vi "trigger-test4.vi"() -> ()   [LabVIEW 2020]
uses:
  Realization/PI650 VoltageAmp/TypeDefs/Channel gain.ctl
  Realization/PIPX40 Matrix/PIPX40 Matrix.lvclass
  Realization/PI650 VoltageAmp/PI650 VoltageAmp.lvclass
  Realization/PI650 VoltageAmp/TypeDefs/Channel DC offset.ctl
  Realization/NI PXI Trigger/NI PXI Trigger.lvclass
  Realization/NI PXI Trigger/PXI Trigger config.ctl
  Realization/NI DMM/NI DMM.lvclass
  Realization/NI DMM/TypeDefs/DMM waveform settings.ctl
  <instrlib>/niDMM/nidmm.llb/niDMM Waveform Function.ctl
  Realization/NI DMM/TypeDefs/Trigger settings.ctl
  <instrlib>/niDMM/nidmm.llb/niDMM Trigger.ctl
  <instrlib>/niDMM/nidmm.llb/niDMM Slope.ctl
  Realization/NI Analog Input/NI Analog Input.lvclass
  Realization/NI DAQmx Base/TypeDefs/Channel Config.ctl
  Realization/NI Analog Output/TypeDefs/Timing Config.ctl
  Realization/NI Analog Output/TypeDefs/Trigger Config.ctl
  Realization/NI Analog Output/NI Analog Output.lvclass
  <instrlib>/niDCPower/nidcpower.llb/niDCPower Output Function.ctl
  Realization/PIPX40 Relay/PIPX40 Relay.lvclass
  <vilib>/measure/NI_MABase.lvlib
panel:
  out "relay info":variant
  out "current measurements":dbl[](array[numeric])
  out "voltage measurements":dbl[](array[numeric])
  in  "instrument handle":refnum<k15>="NI_SMU1"
  in  "noise level":dbl=0.05 format="%#_3f"
  in  "signal type":T1(ring)
  in  "Channel gain":T2={"Channel (CH1)"=3, "Gain (x1)"=2} {"Channel (CH1)" items=["CH1"=1, "CH2"=2, "CH3"=3, "CH4"=4, "CH5"=5]; "Gain (x1)" items=["x1"=1, "x2"=2, "x5"=3, "x7"=4, "x10"=5, "x14"=6, "x20"=7]}
  out "Amp Info":variant
  out "Mx infos":variant[](array[variant])
  out "Waveform Graph":dynamicdata(graph)
  out "error out":errorcluster
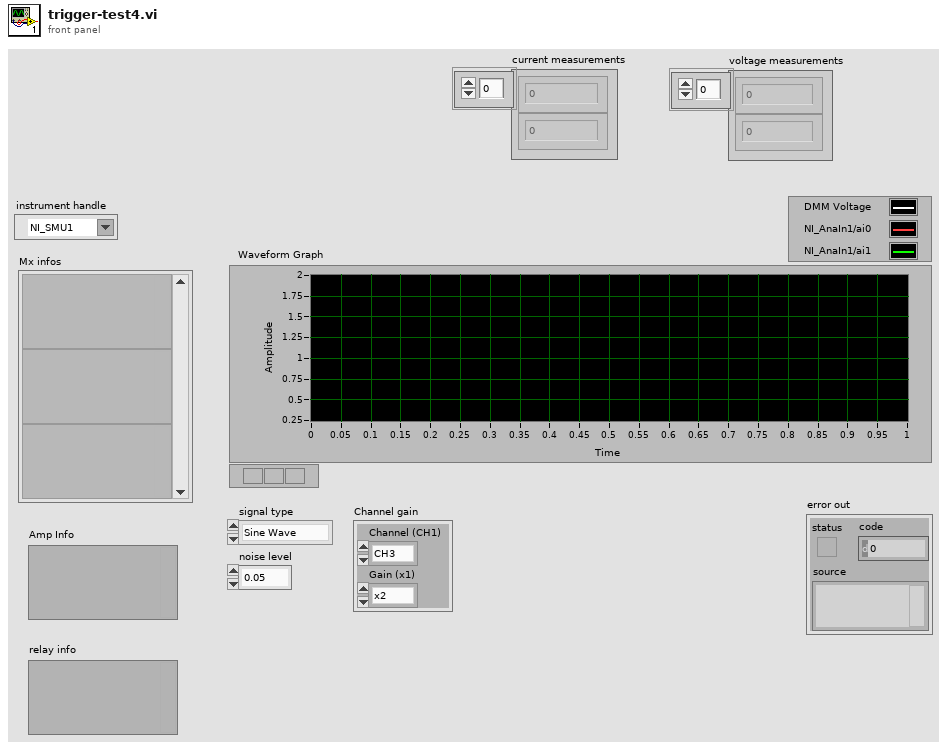
[diagram p1: front panel]
types:
  T1 = enum16{"Sine Wave", "Triangle Wave", "Square Wave", "Sawtooth Wave"}
  T2 = typedef "Channel gain.ctl" = cluster{"Channel (CH1)":u32, "Gain (x1)":u32}
  T3 = typedef "niDCPower Output Function.ctl" = i32
  T4 = typedef "Trigger Config.ctl" = cluster{"trigger type":string, "source":string, "slope":i32, "analog level":dbl, "analog hysteresis":dbl}
  T5 = typedef "Timing Config.ctl" = cluster{"sample mode":i32, "samples per channel":i32, "rate":dbl, "source":string, "active edge":i32}
  T6 = typedef "Channel Config.ctl" = cluster{"channels":string, "maximum value":dbl, "minimum value":dbl, "output terminal configuration":i32, "units":i32}
  T7 = typedef "Trigger settings.ctl" = cluster{"Trigger Source":T8, "Trigger Delay (sec)":dbl, "Slope":T9}
  T8 = typedef "niDMM Trigger.ctl" = enum16{"Immediate", "External", "TTL 0", "TTL 1", "TTL 2", "TTL 3", "TTL 4", "TTL 5", "TTL 6", "Software", "TTL 7", "PXI Star", "LBR Trig 1", "Aux Trig 1"}
  T9 = typedef "niDMM Slope.ctl" = enum16{"Rising Edge", "Falling Edge"}
  T10 = typedef "DMM waveform settings.ctl" = cluster{"Waveform Points":i32, "Function":T11, "Rate":dbl, "Range":dbl, "Settle Time":dbl}
  T11 = typedef "niDMM Waveform Function.ctl" = i32
  T12 = typedef "PXI Trigger config.ctl" = cluster{"counter output":string, "source terminal":string, "destination terminal":string}
  T13 = typedef "Channel DC offset.ctl" = cluster{"Channel (CH1)":u32, "Offset (128)":u32}
  T14 = map{string, refnum<class "PIPX40 Matrix.lvclass">}
  T15 = cluster{"samples per channel":dbl, "samples per channel":dbl}
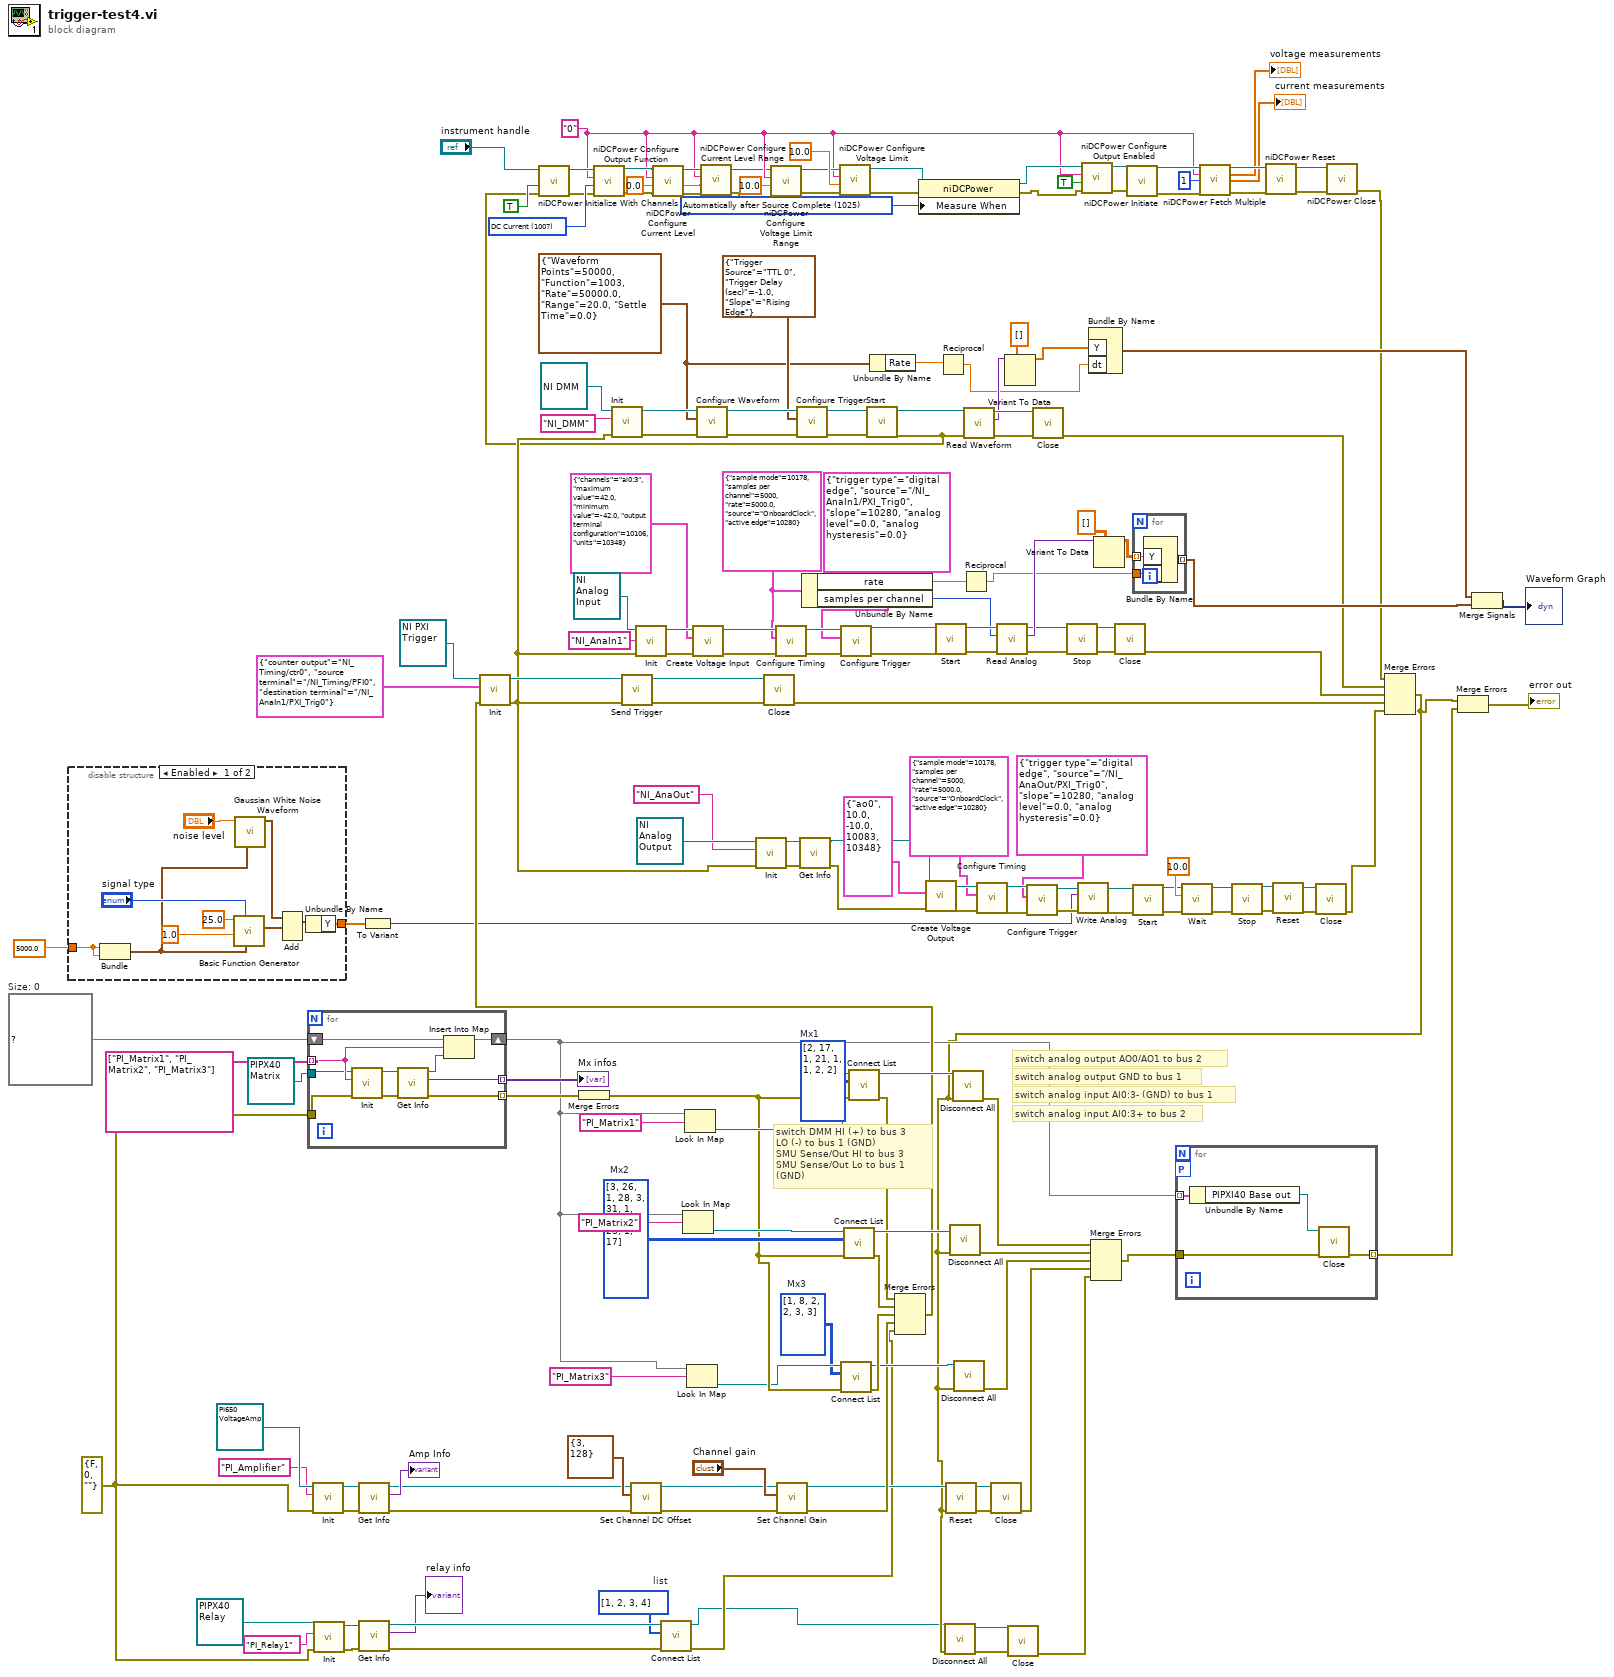
[diagram p0: block diagram]
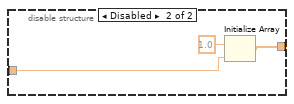
[diagram p2: hidden frame]
diagram:
  w6 = i32[] [1, 2, 3, 4]  # list
  w26 = 1025 items=["Automatically after Source Complete"=1025, "On Demand"=1026, "On Measure Trigger"=1027] ("Measurement:Advanced:Measure When")
  w18 = 0.0 ("current level")
  w19 = "0" ("channel name")
  w50 = T3 1007 items=["DC Voltage"=1006, "DC Current"=1007, "Pulse Voltage"=1049, "Pulse Current"=1050] ("output function")
  w83 = T5 {"sample mode"=10178, "samples per channel"=5000, "rate"=5000.0, "source"="OnboardClock", "active edge"=10280}
  w111 = T10 {"Waveform Points"=50000, "Function"=1003, "Rate"=50000.0, "Range"=20.0, "Settle Time"=0.0}
  w5 = errorcluster {"status"=FALSE, "code"=0, "source"=""} ("error in (no error)")
  w153 = i32[][] [[1, 8], [2, 2], [3, 3]]  # Mx3
  w164 = T14 {}  # Size: 0
  w173 = i32[][] [[3, 26], [1, 28], [3, 31], [1, 19], [3, 23], [1, 17]]  # Mx2
  w175 = i32[][] [[2, 17], [1, 21], [1, 1], [2, 2]]  # Mx1
  # "switch analog input AI0:3+ to bus 2"
  # "switch analog input AI0:3- (GND) to bus 1"
  # "switch analog output GND to bus 1"
  # "switch analog output AO0/AO1 to bus 2"
  # "switch DMM HI (+) to bus 3 \nLO (-) to bus 1 (GND)\nSMU Sense/Out HI to bus 3\nSMU Sense/Out Lo to bus 1 (GND)"
  n1 = disable-structure shown="Enabled" {
    disable-tunnel: 5000.0 ("samples per channel") -> [w189 w192]
    disable-tunnel: [w188 w194] -> w133
    frame Enabled {
      n2 = Bundle("samples per channel"=w189, "samples per channel"=w189) -> (w186:T15)  [unwired: 1 in]
      n3 = call <vilib>:"Basic Function Generator.vi"("sampling info"=w186, "signal type"="signal type", "amplitude"=1.0, "frequency"=25.0) -> ("signal out"=w185:waveform(dbl))  [unwired: 5 in, 2 out]
      n4 = call <vilib>:"Gaussian White Noise Waveform.vi"("sampling info"=w186, "standard deviation"="noise level") -> ("signal out"=w184:waveform(dbl))  [unwired: 8 in, 1 out]
      n5 = Add(1:w185, 2:w184) -> (0:w183:waveform(dbl))  [unwired: 1 in, 1 out]
      n6 = Unbundle By Name(w183) -> ("Y"=w188:dbl[])
    }
    frame Disabled {
      n7 = Initialize Array(1.0 ("element"), w192) -> (w194:dbl[])
    }
  }
  n8 = for {
    tunnel: string[] ["PI_Matrix1", "PI_Matrix2", "PI_Matrix3"] -> [w200] mode=indexing
    tunnel: [w203] -> w178 mode=indexing
    tunnel: [w202] -> w177 mode=indexing
    shift-right: [w201] -> w156
    shift-left: w164 -> [w198]
    tunnel: refnum<class "PIPX40 Matrix.lvclass"> refnum ("PIPXI40 Matrix in") -> [w196]
    tunnel: w5 -> [w195]
    n9 = call-dynamic "Init.vi"("error in (no error)"=w195, "Params"=w200, "PIPXI40 Base in"=w196) -> ("error out"=w204:errorcluster, "PIPXI40 Base out"=w199:refnum<class "PIPX40 Matrix.lvclass">)  [unwired: 7 in]
    n10 = call-dynamic "Get Info.vi"("error in (no error)"=w204, "PIPXI40 Base in"=w199) -> ("error out"=w203:errorcluster, "Info"=w202:variant, "PIPXI40 Base out"=w197:refnum<class "PIPX40 Matrix.lvclass">)  [unwired: 7 in]
    n11 = Insert Into Map(map in=w198, key=w200, value=w197) -> (map out=w201:T14)  [unwired: 2 out]
  }
  "Mx infos" <- w177
  n12 = call-dynamic "Init.vi"("error in (no error)"=w5, "Params"="PI_Amplifier" ("String"), "PI650 VoltageAmp in"=refnum<class "PI650 VoltageAmp.lvclass"> refnum) -> ("error out"=w147:errorcluster, "PI650 VoltageAmp out"=w148:refnum<class "PI650 VoltageAmp.lvclass">)  [unwired: 7 in]
  n13 = call-dynamic "Init.vi"("error in (no error)"=w5, "Params"="PI_Relay1" ("String"), "PIPXI40 Base in"=refnum<class "PIPX40 Relay.lvclass"> refnum ("Pickering.lvlib:PIPX40 Relay.lvclass")) -> ("error out"=w15:errorcluster, "PIPXI40 Base out"=w12:refnum<class "PIPX40 Relay.lvclass">)  [unwired: 7 in]
  n14 = call-dynamic "Get Info.vi"("error in (no error)"=w147, "PI650 VoltageAmp in"=w148) -> ("error out"=w142:errorcluster, "Info"=→"Amp Info":variant, "PI650 VoltageAmp out"=w141:refnum<class "PI650 VoltageAmp.lvclass">)  [unwired: 7 in]
  n15 = call-dynamic "Get Info.vi"("error in (no error)"=w15, "PIPXI40 Base in"=w12) -> ("error out"=w9:errorcluster, "Info"=→"relay info":variant, "PIPXI40 Base out"=w11:refnum<class "PIPX40 Relay.lvclass">)  [unwired: 7 in]
  n16 = To Variant(anything=w133) -> (Variant=w53:variant)
  n17 = Merge Errors(w178) -> (w155:errorcluster)
  n18 = call-dynamic "Set Channel DC Offset.vi"("error in (no error)"=w142, "Params"=T13 {"Channel (CH1)"=3, "Offset (128)"=128}, "PI650 VoltageAmp in"=w141) -> ("error out"=w139:errorcluster, "PI650 VoltageAmp out"=w140:refnum<class "PI650 VoltageAmp.lvclass">)  [unwired: 7 in]
  n19 = call-dynamic "Connect List.vi"("error in (no error)"=w9, "Params"=w6, "PIPXI40 Switching in"=w11) -> ("error out"=w2:errorcluster, "PIPXI40 Switching out"=w1:refnum<class "PIPX40 Relay.lvclass">)  [unwired: 7 in]
  n20 = Look In Map(map=w156, key="PI_Matrix2" ("String")) -> (value=w166:refnum<class "PIPX40 Matrix.lvclass">)  [unwired: 1 in, 1 out]
  n21 = Look In Map(map=w156, key="PI_Matrix1" ("String")) -> (value=w167:refnum<class "PIPX40 Matrix.lvclass">)  [unwired: 1 in, 1 out]
  n22 = Look In Map(map=w156, key="PI_Matrix3" ("String")) -> (value=w154:refnum<class "PIPX40 Matrix.lvclass">)  [unwired: 1 in, 1 out]
  n23 = call-dynamic "Set Channel Gain.vi"("error in (no error)"=w139, "Params"="Channel gain", "PI650 VoltageAmp in"=w140) -> ("error out"=w138:errorcluster, "PI650 VoltageAmp out"=w135:refnum<class "PI650 VoltageAmp.lvclass">)  [unwired: 7 in]
  n24 = Unbundle By Name(w83) -> ("rate"=w81:dbl, "samples per channel"=w82:i32)
  n25 = call-dynamic "Connect List.vi"("error in (no error)"=w155, "Params"=w153, "PIPXI40 Matrix in"=w154) -> ("error out"=w152:errorcluster, "PIPXI40 Matrix out"=w151:refnum<class "PIPX40 Matrix.lvclass">)  [unwired: 7 in]
  n26 = call-dynamic "Connect List.vi"("error in (no error)"=w155, "Params"=w173, "PIPXI40 Matrix in"=w166) -> ("error out"=w162:errorcluster, "PIPXI40 Matrix out"=w171:refnum<class "PIPX40 Matrix.lvclass">)  [unwired: 7 in]
  n27 = call-dynamic "Connect List.vi"("error in (no error)"=w155, "Params"=w175, "PIPXI40 Matrix in"=w167) -> ("error out"=w163:errorcluster, "PIPXI40 Matrix out"=w172:refnum<class "PIPX40 Matrix.lvclass">)  [unwired: 7 in]
  n28 = Unbundle By Name(w111) -> ("Rate"=w110:dbl)
  n29 = Merge Errors(w163, w162, w152, w138, w2) -> (w161:errorcluster)
  n30 = call-dynamic "Init.vi"("error in (no error)"=w161, "Params"=T12 {"counter output"="NI_Timing/ctr0", "source terminal"="/NI_Timing/PFI0", "destination terminal"="/NI_AnaIn1/PXI_Trig0"} ("Cluster of class private data"), "NI PXI Trigger in"=refnum<class "NI PXI Trigger.lvclass"> refnum) -> ("error out"=w25:errorcluster, "NI PXI Trigger out"=w130:refnum<class "NI PXI Trigger.lvclass">)  [unwired: 7 in]
  n31 = call-dynamic "Init.vi"("error in (no error)"=w25, "Params"="NI_DMM", "NI DMM in"=refnum<class "NI DMM.lvclass"> refnum) -> ("error out"=w125:errorcluster, "NI DMM out"=w126:refnum<class "NI DMM.lvclass">)  [unwired: 7 in]
  n32 = call-dynamic "Send Trigger.vi"("error in (no error)"=w25, "NI PXI Trigger in"=w130) -> ("error out"=w129:errorcluster, "NI PXI Trigger out"=w128:refnum<class "NI PXI Trigger.lvclass">)  [unwired: 8 in]
  n33 = call-dynamic "Init.vi"("error in (no error)"=w25, "Params"="NI_AnaIn1" ("String"), "DAQmx Base in"=refnum<class "NI Analog Input.lvclass"> refnum ("NI Analog Input in")) -> ("error out"=w103:errorcluster, "DAQmx Base out"=w102:refnum<class "NI Analog Input.lvclass">)  [unwired: 7 in]
  n34 = call-dynamic "Create Voltage Input.vi"("error in (no error)"=w103, "Params"=T6 {"channels"="ai0:3", "maximum value"=42.0, "minimum value"=-42.0, "output terminal configuration"=10106, "units"=10348} ("Channel Config"), "NI Analog Input in"=w102) -> ("error out"=w104:errorcluster, "NI Analog Input out"=w101:refnum<class "NI Analog Input.lvclass">)  [unwired: 7 in]
  n35 = call-dynamic "Configure Waveform.vi"("error in (no error)"=w125, "Params"=w111, "NI DMM in"=w126) -> ("error out"=w121:errorcluster, "NI DMM out"=w122:refnum<class "NI DMM.lvclass">)  [unwired: 7 in]
  n36 = call-dynamic "Init.vi"("error in (no error)"=w25, "Params"="NI_AnaOut" ("String"), "DAQmx Base in"=refnum<class "NI Analog Output.lvclass"> refnum ("NI DAQmx.lvlib:NI Analog Output.lvclass")) -> ("error out"=w77:errorcluster, "DAQmx Base out"=w78:refnum<class "NI Analog Output.lvclass">)  [unwired: 7 in]
  n37 = call-dynamic "Close.vi"("error in (no error)"=w129, "NI PXI Trigger in"=w128) -> ("error out"=w107:errorcluster)  [unwired: 8 in, 1 out]
  n38 = call-dynamic "Configure Timing.vi"("error in (no error)"=w104, "Params"=w83, "NI DAQmx Base in"=w101) -> ("error out"=w99:errorcluster, "NI DAQmx Base out"=w100:refnum<class "NI Analog Input.lvclass">)  [unwired: 7 in]
  n39 = call-dynamic "Configure Trigger.vi"("error in (no error)"=w121, "Params"=T7 {"Trigger Source"=enum."TTL 0", "Trigger Delay (sec)"=-1.0, "Slope"=enum."Rising Edge"}, "NI DMM in"=w122) -> ("error out"=w119:errorcluster, "NI DMM out"=w120:refnum<class "NI DMM.lvclass">)  [unwired: 7 in]
  n40 = call-dynamic "Get Info.vi"("error in (no error)"=w77, "DAQmx Base in"=w78) -> ("error out"=w54:errorcluster, "DAQmx Base out"=w74:refnum<class "NI Analog Output.lvclass">)  [unwired: 7 in, 1 out]
  n41 = call-dynamic "Configure Trigger.vi"("error in (no error)"=w99, "Params"=T4 {"trigger type"="digital edge", "source"="/NI_AnaIn1/PXI_Trig0", "slope"=10280, "analog level"=0.0, "analog hysteresis"=0.0}, "NI DAQmx Base in"=w100) -> ("error out"=w93:errorcluster, "NI DAQmx Base out"=w92:refnum<class "NI Analog Input.lvclass">)  [unwired: 7 in]
  n42 = call-dynamic "Start.vi"("error in (no error)"=w119, "DMM in"=w120) -> ("error out"=w22:errorcluster, "DMM out"=w118:refnum<class "NI DMM.lvclass">)  [unwired: 8 in]
  n43 = call <instrlib>:"niDCPower Initialize With Channels.vi"("error in (no error)"=w22, "reset (false)"=TRUE, "resource name"="instrument handle") -> ("error out"=w49:errorcluster, "instrument handle out"=w51:refnum<k15>)  [unwired: 7 in]
  n44 = call <instrlib>:"niDCPower Configure Output Function.vi"("error in (no error)"=w49, "output function"=w50, "channel name"=w19, "instrument handle"=w51) -> ("error out"=w47:errorcluster, "instrument handle out"=w48:refnum<k15>)  [unwired: 6 in]
  n45 = call <instrlib>:"niDCPower Configure Current Level.vi"("error in (no error)"=w47, "current level"=w18, "channel name"=w19, "instrument handle"=w48) -> ("error out"=w21:errorcluster, "instrument handle out"=w20:refnum<k15>)  [unwired: 6 in]
  n46 = call <instrlib>:"niDCPower Configure Current Level Range.vi"("error in (no error)"=w21, "current level range"=w18, "channel name"=w19, "instrument handle"=w20) -> ("error out"=w17:errorcluster, "instrument handle out"=w16:refnum<k15>)  [unwired: 6 in]
  n47 = call <instrlib>:"niDCPower Configure Voltage Limit Range.vi"("error in (no error)"=w17, "voltage limit range"=10.0, "channel name"=w19, "instrument handle"=w16) -> ("error out"=w40:errorcluster, "instrument handle out"=w41:refnum<k15>)  [unwired: 6 in]
  n48 = call <instrlib>:"niDCPower Configure Voltage Limit.vi"("error in (no error)"=w40, "voltage limit"=10.0, "channel name"=w19, "instrument handle"=w41) -> ("error out"=w30:errorcluster, "instrument handle out"=w28:refnum<k15>)  [unwired: 6 in]
  n49 = property class="niDCPower"(reference=w28, error in=w30, "Measure When"=w26) -> (reference out=w27:refnum<k15>, error out=w29:errorcluster)
  n50 = call-dynamic "Create Voltage Output.vi"("error in (no error)"=w54, "Params"=T6 {"channels"="ao0", "maximum value"=10.0, "minimum value"=-10.0, "output terminal configuration"=10083, "units"=10348} ("Channel Config"), "NI Analog Output in"=w74) -> ("error out"=w73:errorcluster, "NI Analog Output out"=w72:refnum<class "NI Analog Output.lvclass">)  [unwired: 7 in]
  n51 = call-dynamic "Start.vi"("error in (no error)"=w93, "NI DAQmx Base in"=w92) -> ("error out"=w94:errorcluster, "NI DAQmx Base out"=w91:refnum<class "NI Analog Input.lvclass">)  [unwired: 8 in]
  n52 = Reciprocal(x=w110) -> (1/x=w109:dbl)
  n53 = Reciprocal(x=w81) -> (1/x=w80:dbl)
  n54 = call-dynamic "Read Waveform.vi"("error in (no error)"=w22, "NI DMM in"=w118) -> ("error out"=w116:errorcluster, "Data"=w114:variant, "NI DMM out"=w115:refnum<class "NI DMM.lvclass">)  [unwired: 7 in]
  n55 = call-dynamic "Configure Timing.vi"("error in (no error)"=w73, "Params"=T5 {"sample mode"=10178, "samples per channel"=5000, "rate"=5000.0, "source"="OnboardClock", "active edge"=10280}, "NI DAQmx Base in"=w72) -> ("error out"=w59:errorcluster, "NI DAQmx Base out"=w58:refnum<class "NI Analog Output.lvclass">)  [unwired: 7 in]
  n56 = call-dynamic "Read Analog.vi"("error in (no error)"=w94, "Params"=w82, "NI Analog Input in"=w91) -> ("error out"=w86:errorcluster, "Data"=w89:variant, "NI Analog Input out"=w87:refnum<class "NI Analog Input.lvclass">)  [unwired: 6 in]
  n57 = Variant To Data(type=dbl[] [], Variant=w114) -> (data=w112:dbl[])  [unwired: 1 in, 1 out]
  n58 = call-dynamic "Configure Trigger.vi"("error in (no error)"=w59, "Params"=T4 {"trigger type"="digital edge", "source"="/NI_AnaOut/PXI_Trig0", "slope"=10280, "analog level"=0.0, "analog hysteresis"=0.0}, "NI DAQmx Base in"=w58) -> ("error out"=w56:errorcluster, "NI DAQmx Base out"=w57:refnum<class "NI Analog Output.lvclass">)  [unwired: 7 in]
  n59 = call-dynamic "Close.vi"("error in (no error)"=w116, "NI DMM in"=w115) -> ("error out"=w105:errorcluster)  [unwired: 8 in, 1 out]
  n60 = call-dynamic "Stop.vi"("error in (no error)"=w86, "NI DAQmx Base in"=w87) -> ("error out"=w85:errorcluster, "NI DAQmx Base out"=w88:refnum<class "NI Analog Input.lvclass">)  [unwired: 8 in]
  n61 = call-dynamic "Write Analog.vi"("error in (no error)"=w56, "Params"=w53, "NI Analog Output in"=w57) -> ("error out"=w70:errorcluster, "NI Analog Output out"=w69:refnum<class "NI Analog Output.lvclass">)  [unwired: 7 in]
  n62 = call <instrlib>:"niDCPower Configure Output Enabled.vi"("error in (no error)"=w29, "output enabled"=TRUE, "channel name"=w19, "instrument handle"=w27) -> ("error out"=w36:errorcluster, "instrument handle out"=w35:refnum<k15>)  [unwired: 6 in]
  n63 = Bundle By Name("Y"=w112, "dt"=w109) -> (w108:waveform(dbl))  [unwired: 1 in]
  n64 = Variant To Data(type=dbl[][] [], Variant=w89) -> (data=w84:dbl[][])  [unwired: 1 in, 1 out]
  n65 = call-dynamic "Close.vi"("error in (no error)"=w85, "DAQmx Base in"=w88) -> ("error out"=w106:errorcluster)  [unwired: 8 in, 1 out]
  n66 = call <instrlib>:"niDCPower Initiate.vi"("error in (no error)"=w36, "instrument handle"=w35) -> ("error out"=w43:errorcluster, "instrument handle out"=w42:refnum<k15>)  [unwired: 2 in, 6 out]
  n67 = for {
    tunnel: w84 -> [w207] mode=indexing
    tunnel: [w206] -> w132 mode=indexing
    tunnel: w80 -> [w205]
    n68 = Bundle By Name("Y"=w207, "dt"=w205) -> (w206:waveform(dbl))  [unwired: 1 in]
  }
  n69 = call-dynamic "Start.vi"("error in (no error)"=w70, "NI DAQmx Base in"=w69) -> ("error out"=w63:errorcluster, "NI DAQmx Base out"=w62:refnum<class "NI Analog Output.lvclass">)  [unwired: 8 in]
  n70 = call-dynamic "Wait.vi"("error in (no error)"=w63, "Params"=10.0, "NI DAQmx Base in"=w62) -> ("error out"=w65:errorcluster, "NI DAQmx Base out"=w66:refnum<class "NI Analog Output.lvclass">)  [unwired: 7 in]
  n71 = call <instrlib>:"niDCPower Fetch Multiple.vi"("instrument handle"=w42, "channel name"=w19, "count (1)"=1, "error in (no error)"=w43) -> ("instrument handle out"=w37:refnum<k15>, "voltage measurements"=→"voltage measurements":dbl[], "current measurements"=→"current measurements":dbl[], "error out"=w38:errorcluster)  [unwired: 6 in, 2 out]
  n72 = call-dynamic "Stop.vi"("error in (no error)"=w65, "NI DAQmx Base in"=w66) -> ("error out"=w68:errorcluster, "NI DAQmx Base out"=w67:refnum<class "NI Analog Output.lvclass">)  [unwired: 8 in]
  n73 = call <instrlib>:"niDCPower Reset.vi"("error in (no error)"=w38, "instrument handle"=w37) -> ("error out"=w45:errorcluster, "instrument handle out"=w44:refnum<k15>)  [unwired: 8 in]
  n74 = call-dynamic "Reset.vi"("error in (no error)"=w68, "DAQmx Base in"=w67) -> ("error out"=w61:errorcluster, "DAQmx Base out"=w60:refnum<class "NI Analog Output.lvclass">)  [unwired: 8 in]
  n75 = call-dynamic "Close.vi"("error in (no error)"=w61, "DAQmx Base in"=w60) -> ("error out"=w180:errorcluster)  [unwired: 8 in, 1 out]
  n76 = call <instrlib>:"niDCPower Close.vi"("error in (no error)"=w45, "instrument handle"=w44) -> ("error out"=w24:errorcluster)  [unwired: 9 in]
  n77 = Merge Errors(w24, w105, w106, w107, w180) -> (w4:errorcluster)
  n78 = call-dynamic "Disconnect All.vi"("error in (no error)"=w4, "PIPXI40 Switching in"=w1) -> ("error out"=w7:errorcluster, "PIPXI40 Switching out"=w8:refnum<class "PIPX40 Relay.lvclass">)  [unwired: 8 in]
  n79 = call-dynamic "Reset.vi"("error in (no error)"=w4, "PI650 VoltageAmp in"=w135) -> ("error out"=w136:errorcluster, "PI650 VoltageAmp out"=w137:refnum<class "PI650 VoltageAmp.lvclass">)  [unwired: 8 in]
  n80 = call-dynamic "Disconnect All.vi"("error in (no error)"=w4, "PIPXI40 Matrix in"=w171) -> ("error out"=w170:errorcluster)  [unwired: 8 in, 1 out]
  n81 = call-dynamic "Disconnect All.vi"("error in (no error)"=w4, "PIPXI40 Matrix in"=w172) -> ("error out"=w169:errorcluster)  [unwired: 8 in, 1 out]
  n82 = call-dynamic "Disconnect All.vi"("error in (no error)"=w4, "PIPXI40 Matrix in"=w151) -> ("error out"=w150:errorcluster)  [unwired: 8 in, 1 out]
  n83 = call-dynamic "Close.vi"("error in (no error)"=w136, "PI650 VoltageAmp in"=w137) -> ("error out"=w134:errorcluster)  [unwired: 8 in, 1 out]
  n84 = call-dynamic "Close.vi"("error in (no error)"=w7, "PIPXI40 Base in"=w8) -> ("error out"=w3:errorcluster)  [unwired: 8 in, 1 out]
  n85 = Merge Errors(w169, w170, w150, w134, w3) -> (w168:errorcluster)
  n86 = for {
    tunnel: w168 -> [w210]
    tunnel: [w211] -> w160 mode=indexing
    workers-P: _ -> [_]
    tunnel: w156 -> [w209] mode=indexing
    n87 = Unbundle By Name(w209) -> ("PIPXI40 Base out"=w208:refnum<class "PIPX40 Matrix.lvclass">)
    n88 = call-dynamic "Close.vi"("error in (no error)"=w210, "PIPXI40 Base in"=w208) -> ("error out"=w211:errorcluster)  [unwired: 8 in, 1 out]
  }
  n89 = Merge Errors(w4, w160) -> (→"error out":errorcluster)
  n90 = Merge Signals(w108, w132) -> (→"Waveform Graph":dynamicdata)
